vi "Draw.vi"(8 "error in (no error)":errorcluster, 10 "2D Picture in":picture, 11 "Text in":refnum<class "Text.lvclass">) -> (0 "error out":errorcluster, 2 "2D Picture out":picture, 3 "Text out":refnum<class "Text.lvclass">)   [LabVIEW 2021, in "Picture2D.lvlib" / "Text.lvclass"]
uses:
  Text.lvclass
  Shape/Shape.lvclass
  Color/Color.lvclass
  Font/Font.lvclass
  Point/Point.lvclass
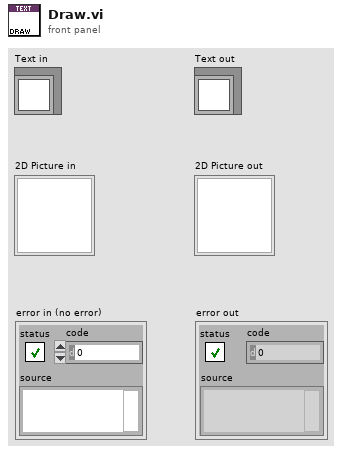
[diagram p1: front panel]
types:
  T1 = cluster{"Font Name:":string, "Size":i16, "Strikeout?":bool, "Italic?":bool, "Underline?":bool, "Outline?":bool, "Shadow?":bool, "Bold?":bool}
  T2 = enum16{"User-specified Font", "Application Font", "System Font", "Dialog Font"}
  T3 = cluster{"horizontal":enum16{"left", "center", "right"}, "vertical":enum16{"top", "center", "bottom"}}
  T4 = enum16{"None", "Stacked", "Clockwise", "Counterclockwise"}
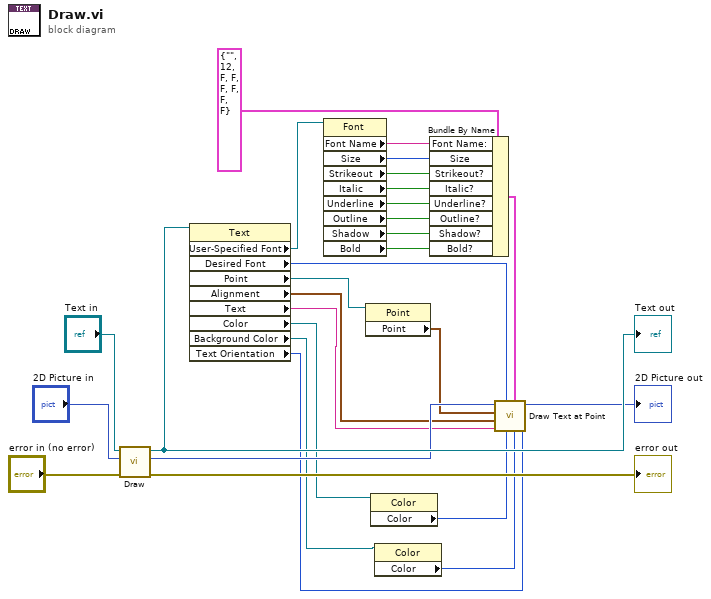
[diagram p0: block diagram]
diagram:
  n1 = call-parent "Draw.vi"("error in (no error)"="error in (no error)", "2D Picture in"="2D Picture in", "Shape in"="Text in") -> ("error out"=→"error out":errorcluster, "2D Picture out"=w23:picture, "Shape out"=w24:refnum<class "Text.lvclass">)  [unwired: 6 in]
  "Text out" <- w24
  n2 = property class="Text"(reference=w24) -> ("User-Specified Font"=w9:refnum<class "Font.lvclass">, "Desired Font"=w21:T2, "Point"=w20:refnum<class "Point.lvclass">, "Alignment"=w19:T3, "Text"=w18:string, "Color"=w17:refnum<class "Color.lvclass">, "Background Color"=w15:refnum<class "Color.lvclass">, "Text Orientation "=w13:T4)  [unwired: 1 in, 2 out]
  n3 = property class="Font"(reference=w9) -> ("Font Name"=w8:string, "Size"=w7:i16, "Strikeout"=w6:bool, "Italic"=w5:bool, "Underline"=w4:bool, "Outline"=w3:bool, "Shadow"=w2:bool, "Bold"=w1:bool)  [unwired: 1 in, 2 out]
  n4 = property class="Point"(reference=w20) -> ("Point"=w12:cluster{"x":i16, "y":i16})  [unwired: 1 in, 2 out]
  n5 = property class="Color"(reference=w17) -> ("Color"=w16:u32)  [unwired: 1 in, 2 out]
  n6 = property class="Color"(reference=w15) -> ("Color"=w14:u32)  [unwired: 1 in, 2 out]
  n7 = Bundle By Name(cluster=T1 {"Font Name:"="", "Size"=12, "Strikeout?"=FALSE, "Italic?"=FALSE, "Underline?"=FALSE, "Outline?"=FALSE, "Shadow?"=FALSE, "Bold?"=FALSE} ("[user-specified font]"), "Font Name:"=w8, "Size"=w7, "Strikeout?"=w6, "Italic?"=w5, "Underline?"=w4, "Outline?"=w3, "Shadow?"=w2, "Bold?"=w1) -> (w10:T1)
  n8 = call <vilib>:"Draw Text at Point.vi"("text orientation"=w13, "BG color(transparent)"=w14, "[user-specified font]"=w10, "text color(black)"=w16, "desired font(Application)"=w21, "text"=w18, "alignment(left, top)"=w19, "origin"=w12, "picture"=w23) -> ("new picture"=→"2D Picture out":picture)  [unwired: 1 in, 1 out]
